vi "TimeArrayToStrings.vi"(1 "quote":bool=TRUE, 2 "Array":timestamp[](array[timestamp])) -> (0 "time strings":string[](array[string]))   [LabVIEW 2013]
doc: "Converts and array of Labview timestamps into a ISO 8601 like time string that is understandable by other programs including web-browsers."
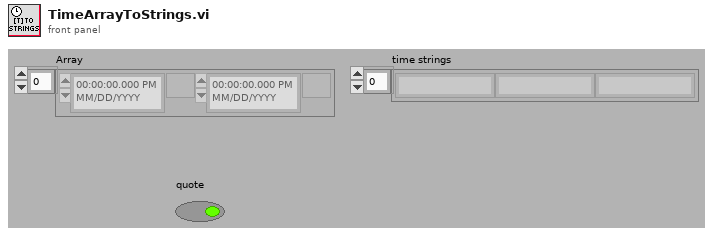
[diagram p1: front panel]
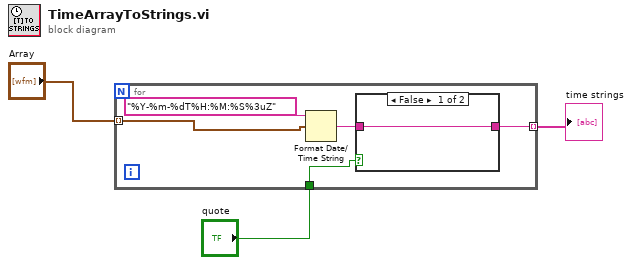
[diagram p0: block diagram]
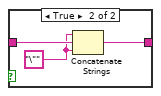
[diagram p2: hidden frame]
diagram:
  n1 = for {
    tunnel: [w4] -> w3 mode=indexing
    tunnel: "Array" -> [w7] mode=indexing
    tunnel: "quote" -> [w6]
    n2 = Format Date/Time String(time format string (%c)="%Y-%m-%dT%H:%M:%S%3uZ", seconds (now)=w7) -> (date/time string=w5:string)  [unwired: 1 in]
    n3 = case shown="False" w6 {
      tunnel: w5 -> [w9 w12]
      tunnel: [w9 w10] -> w4
      frame False {
      }
      frame True {
        w11 = "\""
        n4 = Concatenate Strings(w11, w12, w11) -> (w10:string)
      }
    }
  }
  "time strings" <- w3
